vi "Center Objects.vi"(7 "grid multiplier (6)":u32=6, 8 "error in (no error)":errorcluster, 10 "case structure in":refnum<vi>, 11 "VI in":refnum<vi>) -> (0 "error out":errorcluster, 2 "case structure out":refnum<vi>, 3 "VI out":refnum<vi>)   [LabVIEW 2017]
uses:
  <vilib>/Utility/miscctls.llb/LVBoundsTypeDef.ctl
  <resource>/dialog/lvconfig.llb/LV Config Read Numeric (I32).vi
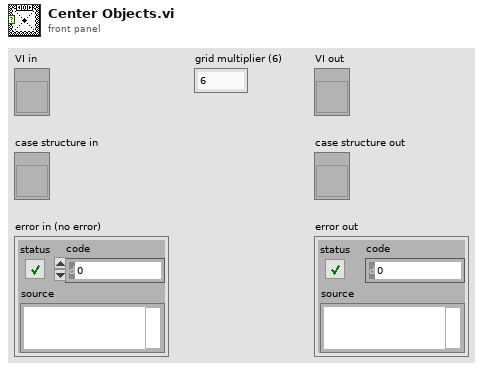
[diagram p1: front panel]
types:
  T1 = typedef "LVBoundsTypeDef.ctl" = cluster{"Width":u32, "Height":u32}
  T2 = cluster{"Left":i16, "Top":i16, "Right":i16, "Bottom":i16}
  T3 = typedef "LVRectTypeDef.ctl" = cluster{"Left":i16, "Top":i16, "Right":i16, "Bottom":i16}
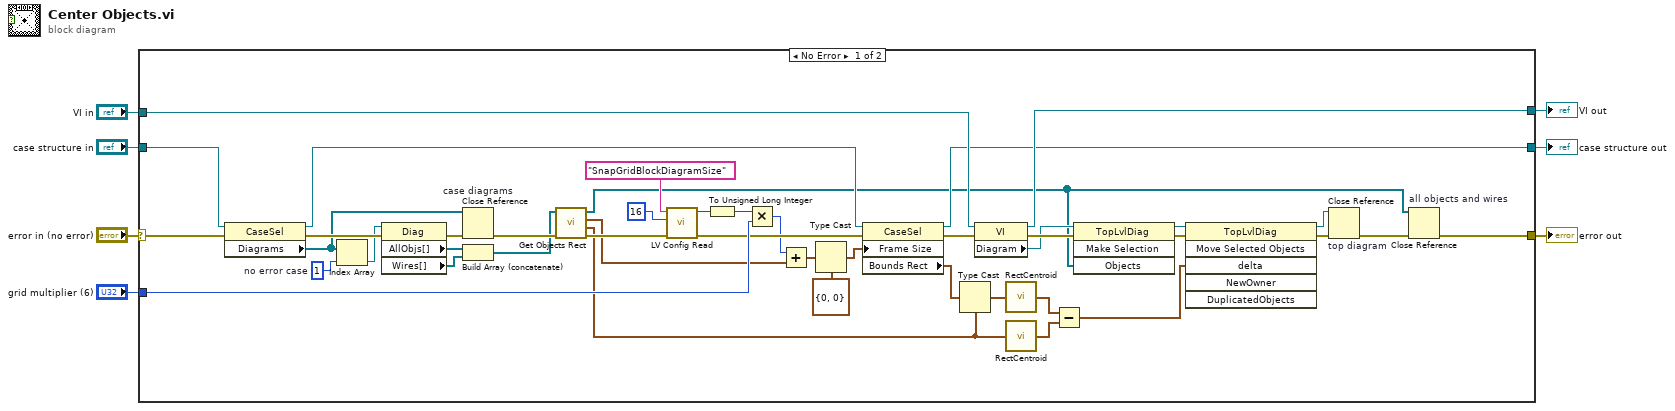
[diagram p0: block diagram]
diagram:
  n1 = case shown="No Error" "error in (no error)" {
    selector: "error in (no error)" -> [w23 w53]
    tunnel: "case structure in" -> [w42 w51]
    tunnel: "VI in" -> [w31 w52]
    tunnel: [w30 w52] -> w5
    tunnel: [w26 w53] -> w4
    tunnel: [w25 w51] -> w3
    tunnel: "grid multiplier (6)" -> [w50 _]
    frame No Error {
      w34 = 1  # no error case
      n2 = property class="CaseSel"(reference=w42, error in=w23) -> (reference out=w43:refnum<vi>, error out=w41:errorcluster, "Diagrams"=w24:refnum<vi>[])
      n3 = Index Array(array=w24, index=w34) -> (element=w38:refnum<vi>)
      n4 = property class="Diag"(reference=w38, error in=w41) -> (error out=w44:errorcluster, "AllObjs[]"=w11:refnum<vi>[], "Wires[]"=w8:refnum<vi>[])  [unwired: 1 out]
      n5 = Close Reference "case diagrams"(reference=w24, error in (no error)=w44) -> (error out=w49:errorcluster)
      n6 = Build Array (concatenate)(w11, w8) -> (w9:refnum<vi>[])
      n7 = call "Get Objects Rect.vi"("error in (no error)"=w49, "objects in"=w9) -> ("error out"=w48:errorcluster, "total bounds rect"=w16:T2, "rect size"=w15:cluster{"Width":u32, "Height":u32}, "objects out"=w10:refnum<vi>[])  [unwired: 6 in]
      n8 = call-poly <resource>:"LV Config Read.vi"("error in"=w48, "default value"=i16 16, "key"="SnapGridBlockDiagramSize") -> ("error out"=w47:errorcluster, "value"=w20:i32)  [unwired: 2 in, 1 out]
      n9 = To Unsigned Long Integer(number=w20) -> (unsigned 32bit integer=w18:u32)
      n10 = Multiply(x=w18, y=w50) -> (x*y=w19:u32)
      n11 = Add(x=w19, y=w15) -> (x+y=w14:cluster{"Width":u32, "Height":u32})
      n12 = Type Cast(type=T1 {"Width"=0, "Height"=0} ("Frame Size"), x=w14) -> (*(type *) &x=w12:T1)
      n13 = property class="CaseSel"(reference=w43, error in=w47, "Frame Size"=w12) -> (reference out=w25:refnum<vi>, error out=w32:errorcluster, "Bounds Rect"=w35:T3)
      n14 = Type Cast(type=w16, x=w35) -> (*(type *) &x=w17:T2)
      n15 = property class="VI"(reference=w31, error in=w32) -> (reference out=w30:refnum<vi>, error out=w46:errorcluster, "Diagram"=w33:refnum<vi>)
      n16 = call <vilib>:"RectCentroid.vi"("rect"=w17) -> ("point"=w36:cluster{"x":i16, "y":i16})
      n17 = call <vilib>:"RectCentroid.vi"("rect"=w16) -> ("point"=w37:cluster{"x":i16, "y":i16})
      n18 = Subtract(x=w36, y=w37) -> (x-y=w40:cluster{"x":i16, "y":i16})
      n19 = invoke class="TopLvlDiag" method="Make Selection"(reference=w33, error in=w46, "Objects"=w10) -> (reference out=w39:refnum<vi>, error out=w45:errorcluster)  [unwired: 1 in, 2 out]
      n20 = invoke class="TopLvlDiag" method="Move Selected Objects"(reference=w39, error in=w45, "delta"=w40) -> (reference out=w28:refnum<vi>, error out=w29:errorcluster)  [unwired: 3 in, 4 out]
      n21 = Close Reference "top diagram"(reference=w28, error in (no error)=w29) -> (error out=w27:errorcluster)
      n22 = Close Reference "all objects and wires"(reference=w10, error in (no error)=w27) -> (error out=w26:errorcluster)
    }
    frame Error {
    }
  }
  "VI out" <- w5
  "error out" <- w4
  "case structure out" <- w3
